vi "Test Draw.vi"(11 "Test Case In":refnum<class "Renderer Tests.lvclass">) -> (0 "error out":errorcluster, 3 "Test Case Out":refnum<class "Renderer Tests.lvclass">)   [LabVIEW 2021, in "Renderer Tests.lvclass"]
uses:
  Renderer Tests.lvclass
  Application Specific/Renderer/Renderer.lvclass/Renderer.ctl
  Application Specific/Texture/Texture.lvclass/Texture.ctl
  Re-use Libraries/Vector 2D/Vector 2D.lvclass/Vector 2D.ctl
  Re-use Libraries/Vector 2D/Vector 2D.lvclass
  Application Specific/Renderer/Renderer.lvclass
  C:/Program Files (x86)/National Instruments/LabVIEW 2026/vi.lib/Astemes/LUnit/Test Case.lvclass
  Application Specific/Texture/Texture.lvclass
  <vilib>/picture/picture.llb/Draw True-Color Pixmap.vi
  LabSDL2/Source/Libraries/LibSDL2 Wrapper/Controls/Rectangle.ctl
  LabSDL2/Source/Libraries/LibSDL2 Wrapper/LibSDL2.lvlib
  <vilib>/Astemes/LUnit/Test Case.lvclass
panel:
  out "Similar Ratio":dbl
  out "2D Picture":picture
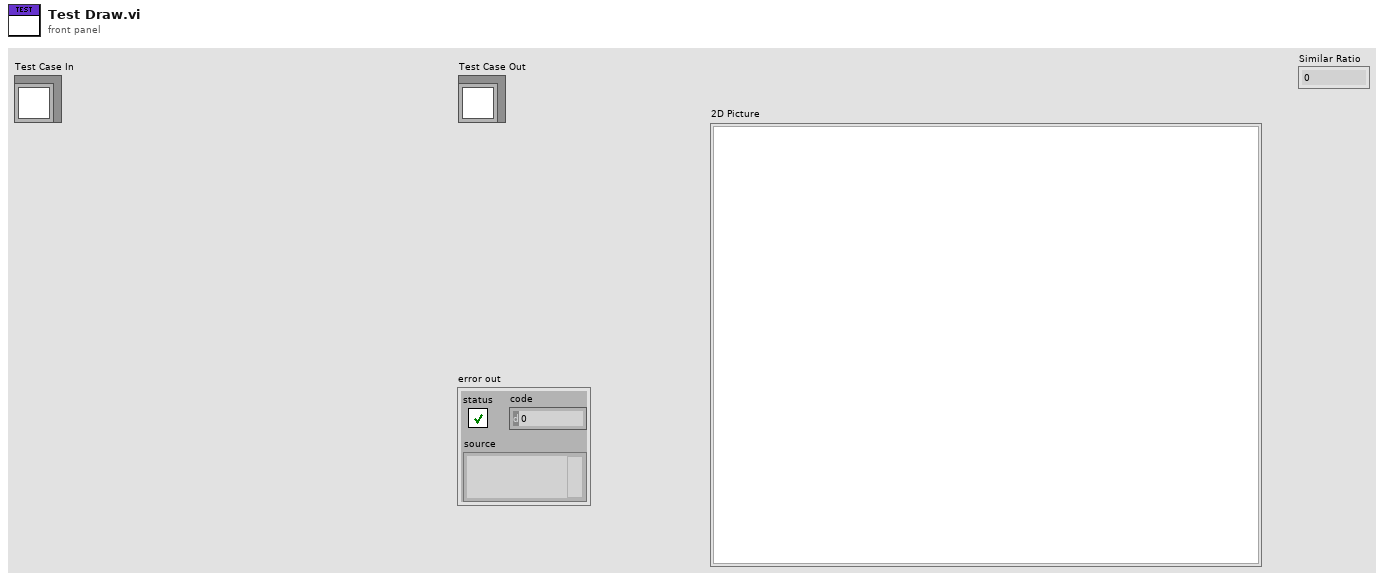
[diagram p1: front panel]
types:
  T1 = cluster{"left":i16, "top":i16, "right":i16, "bottom":i16}
  T2 = typedef "LibSDL2.lvlib/Rectangle.ctl" = cluster{"x":i32, "y":i32, "Width":i32, "Height":i32}
  T3 = typedef "imagedata.ctl" = cluster{"image type":i32, "image depth":i32, "image":u8[], "mask":u8[], "colors":u32[], "Rectangle":cluster{"left":i16, "top":i16, "right":i16, "bottom":i16}}
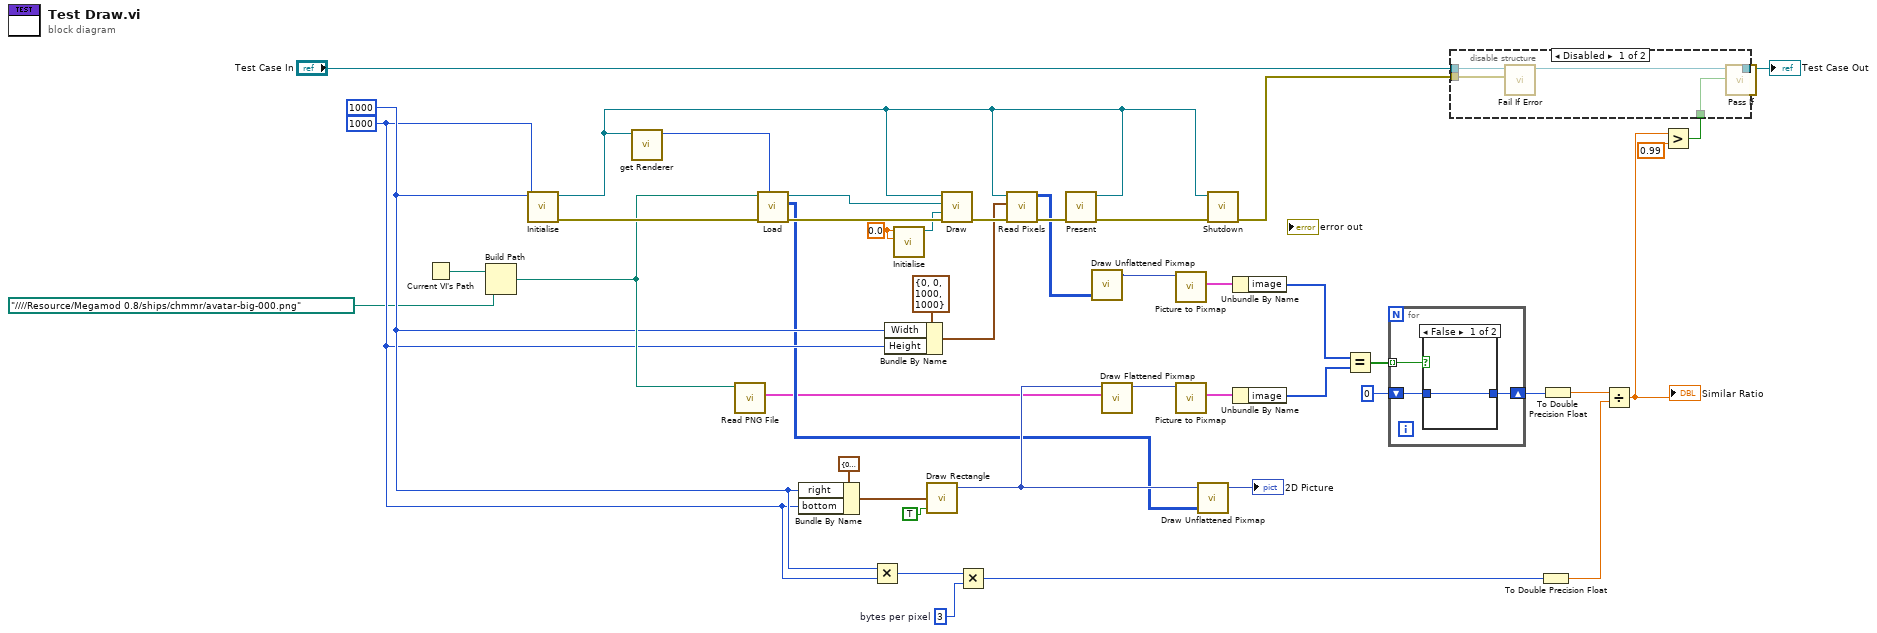
[diagram p0: block diagram]
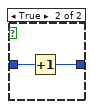
[diagram p3: hidden frame]
diagram:
  w7 = sgl 0.0 ("x")
  w13 = 3  # bytes per pixel
  w19 = 1000 ("Height")
  w20 = 1000 ("Width")
  n1 = Current VI's Path() -> (path=w41:path)
  n2 = Build Path(base path=w41, name or relative path=path "../../../../Resource/Megamod 0.8/ships/chmmr/avatar-big-000.png" ("Path")) -> (appended path=w32:path)
  n3 = call "Initialise.vi"("Window Height"=w19, "Window Width"=w20) -> ("error out"=w42:errorcluster, "Renderer out"=w40:refnum<class "Renderer.lvclass">)  [unwired: 8 in]
  n4 = call-dynamic "get Renderer.vi"("Renderer in"=w40) -> ("Renderer"=w44:u32)  [unwired: 10 in]
  n5 = call <vilib>:"Read PNG File.vi"("path to PNG file"=w32) -> ("image data"=w2:T3)  [unwired: 8 in, 2 out]
  n6 = call "Load.vi"("Renderer"=w44, "error in (no error)"=w42, "Path"=w32) -> ("error out"=w33:errorcluster, "Pixels"=w3:u32[][], "Texture out"=w43:refnum<class "Texture.lvclass">)  [unwired: 6 in]
  n7 = Bundle By Name(cluster=T1 {"left"=0, "top"=0, "right"=0, "bottom"=0} ("rect"), "right"=w20, "bottom"=w19) -> (w30:T1)
  n8 = Multiply(x=w20, y=w19) -> (x*y=w12:i32)
  n9 = Bundle By Name(cluster=T2 {"x"=0, "y"=0, "Width"=1000, "Height"=1000} ("Rectangle"), "Width"=w20, "Height"=w19) -> (w34:T2)
  n10 = call "Initialise.vi"("y"=w7, "x"=w7) -> ("Vector 2D out"=w8:refnum<class "Vector 2D.lvclass">)  [unwired: 9 in]
  n11 = call <vilib>:"Draw Rectangle.vi"("rect"=w30, "fill?(F)"=TRUE) -> ("new picture"=w5:picture)  [unwired: 7 in]
  n12 = call "Draw.vi"("error in (no error)"=w33, "Destination"=w8, "Texture"=w43, "Renderer"=w40) -> ("error out"=w39:errorcluster)  [unwired: 7 in]
  n13 = Multiply(x=w12, y=w13) -> (x*y=w11:i32)
  n14 = call "Read Pixels.vi"("error in (no error)"=w39, "Rectangle"=w34, "Renderer"=w40) -> ("error out"=w38:errorcluster, "Pixels"=w36:i32[][])  [unwired: 7 in]
  n15 = call "Present.vi"("error in (no error)"=w38, "Renderer"=w40) -> ("error out"=w37:errorcluster)  [unwired: 9 in]
  n16 = call-poly <vilib>:"Draw Unflattened Pixmap.vi"("data (RGB format)"=w36) -> ("new picture"=w6:picture)  [unwired: 8 in]
  n17 = call <vilib>:"Draw Flattened Pixmap.vi"("image data"=w2, "picture"=w5) -> ("new picture"=w28:picture)  [unwired: 7 in]
  n18 = call <vilib>:"Picture to Pixmap.vi"("picture"=w6) -> ("image data"=w26:T3)  [unwired: 9 in, 1 out]
  n19 = call <vilib>:"Picture to Pixmap.vi"("picture"=w28) -> ("image data"=w27:T3)  [unwired: 9 in, 1 out]
  n20 = call-poly <vilib>:"Draw Unflattened Pixmap.vi"("picture"=w5, "data (RGB format)"=w3) -> ("new picture"=→"2D Picture":picture)  [unwired: 7 in]
  n21 = call "Shutdown.vi"("error in (no error)"=w37, "Renderer"=w40) -> ("error out"=w9:errorcluster)  [unwired: 9 in]
  n22 = Unbundle By Name(w26) -> ("image"=w25:u8[])
  n23 = Unbundle By Name(w27) -> ("image"=w24:u8[])
  n24 = Equal?(x=w25, y=w24) -> (x = y?=w23:bool[])
  n25 = for {
    tunnel: w23 -> [w48] mode=indexing
    shift-right: [w46] -> w21
    shift-left: 0 -> [w47]
    n26 = case shown="False" w48 {
      tunnel: w47 -> [w49 w51]
      tunnel: [w49 w50] -> w46
      frame False {
      }
      frame True {
        n27 = Increment(x=w51) -> (x+1=w50:i32)
      }
    }
  }
  n28 = To Double Precision Float(number=w11) -> (double precision float=w17:dbl)
  n29 = To Double Precision Float(number=w21) -> (double precision float=w18:dbl)
  n30 = Divide(x=w18, y=w17) -> (x/y=w16:dbl)
  "Similar Ratio" <- w16
  n31 = Greater?(x=w16, y=0.99) -> (0:w15:bool)
  n32 = disable-structure shown="Disabled" {
    disable-tunnel: [w56 w57] -> w45
    disable-tunnel: w15 -> [w55 _]
    disable-tunnel: "Test Case In" -> [w54 w57]
    disable-tunnel: w9 -> [w52 _]
    frame Disabled {
      n33 = call <vilib>:"Fail If Error.vi"("Assert error"=w52, "LUnit Test Case In"=w54) -> ("LUnit Test Case Out"=w53:refnum<class "Renderer Tests.lvclass">)  [unwired: 8 in, 1 out]
      n34 = call <vilib>:"Pass If.vi"("Pass?"=w55, "LUnit Test Case In"=w53) -> ("LUnit Test Case Out"=w56:refnum<class "Renderer Tests.lvclass">)  [unwired: 8 in, 1 out]
    }
    frame Enabled {
    }
  }
  "Test Case Out" <- w45
